vi "Read_UI2R_from_File.vi"(8 "error in (no error)":errorcluster, 10 "UI2R Save Filepath":path, 11 "UI_Interaction_Manager in":refnum<class "UI_Interaction_Manager.lvclass">) -> (0 "error out":errorcluster, 1 "ControlValueUpdates[]":T1[](array[typedef]), 2 "UI Filepath":path, 3 "UI_Interaction_Manager out":refnum<class "UI_Interaction_Manager.lvclass">)   [LabVIEW 2011, in "UI_Interaction_Manager.lvclass"]
uses:
  UI_Interaction_Manager.lvclass
  TypeDefs/ControlValueUpdate.ctl
  TypeDefs/UI_Interaction_Record.ctl
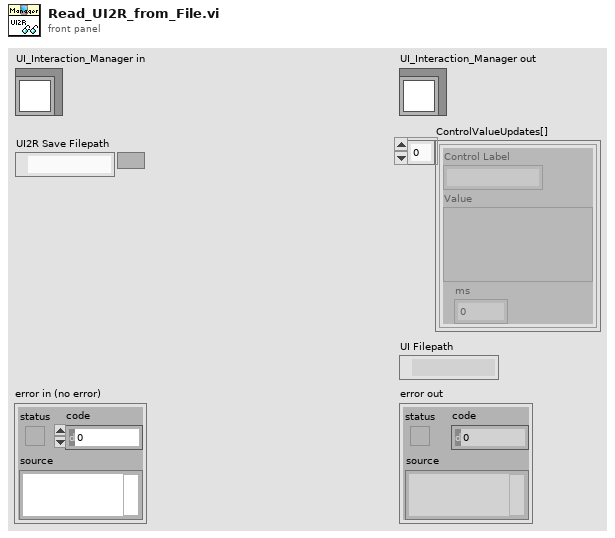
[diagram p1: front panel]
types:
  T1 = typedef "UI_Interaction_Manager.lvclass/ControlValueUpdate.ctl" = cluster{"Control Label":string, "Value":variant, "ms":u32}
  T2 = typedef "UI_Interaction_Manager.lvclass/UI_Interaction_Record.ctl" = cluster{"UI Filepath":path, "Recorded Events":T1[]}
  T3 = enum16{"open", "replace", "create", "open or create", "replace or create", "replace or create with confirmation"}
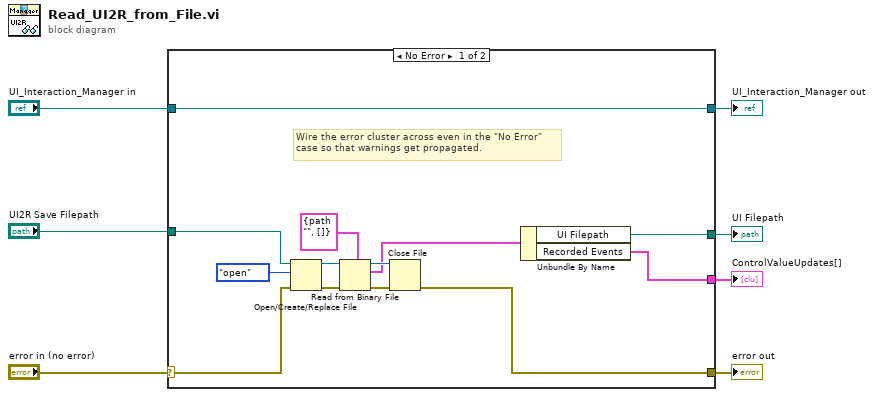
[diagram p0: block diagram]
diagram:
  n1 = case shown="No Error" "error in (no error)" {
    selector: "error in (no error)" -> [w12 w22]
    tunnel: [w8 w22] -> w6
    tunnel: [w20 w21] -> w4
    tunnel: "UI_Interaction_Manager in" -> [w20 w21]
    tunnel: [w14 _] -> w1
    tunnel: "UI2R Save Filepath" -> [w13 _]
    tunnel: [w11 _] -> w2
    frame No Error {
      # "Wire the error cluster across even in the \"No Error\"\ncase so that warnings get propagated."
      n2 = Open/Create/Replace File(file path (use dialog)=w13, error in=w12, operation (0:open)=T3."open") -> (refnum out=w18:refnum<file>, error out=w17:errorcluster)  [unwired: 3 in, 1 out]
      n3 = Read from Binary File(5:T2 {"UI Filepath"=path "", "Recorded Events"=[]} ("Cluster"), 8:w17, 11:w18) -> (0:w16:errorcluster, 2:w9:T2, 3:w15:refnum<file>)  [unwired: 3 in, 1 out]
      n4 = Close File(refnum=w15, error in=w16) -> (error out=w8:errorcluster)  [unwired: 1 out]
      n5 = Unbundle By Name(w9) -> ("UI Filepath"=w11:path, "Recorded Events"=w14:T1[])
    }
    frame Error {
    }
  }
  "error out" <- w6
  "UI_Interaction_Manager out" <- w4
  "ControlValueUpdates[]" <- w1
  "UI Filepath" <- w2
